vi "create.AddOrderShort.vi"(8 "error in (no error)":errorcluster, 10 "AddOrderShort.Parameters":T1, 11 "AddOrderShort in":refnum<class "AddOrderShort.lvclass">) -> (0 "error out":errorcluster, 3 "AddOrderShort out":refnum<class "AddOrderShort.lvclass">)   [LabVIEW 2020, in "AddOrderShort.lvclass"]
uses:
  AddOrderShort.lvclass
  AddOrderShort.Parameters.ctl
  FieldSpec.ctl
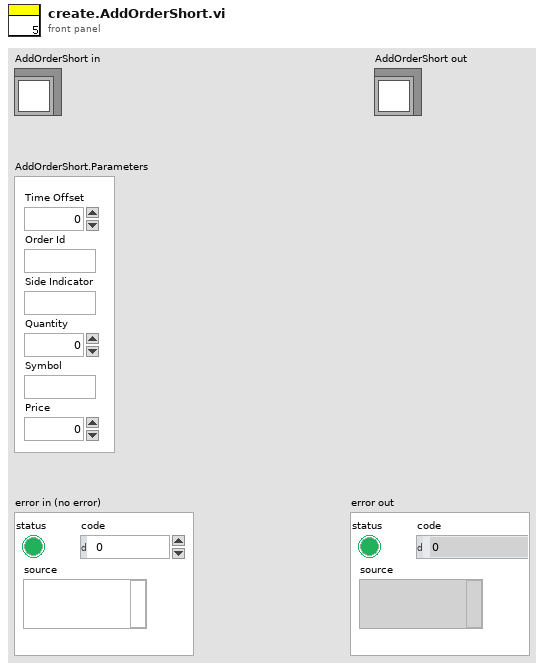
[diagram p1: front panel]
types:
  T1 = typedef "AddOrderShort.lvclass/AddOrderShort.Parameters.ctl" = cluster{"Time Offset":u32, "Order Id":string, "Quantity":u32, "Symbol":string, "Side Indicator":string, "Price":dbl}
  T2 = typedef "FieldSpec.ctl" = cluster{"Name":string, "Offset":i32, "Length":i32, "FieldType":enum16{"Alphanumeric", "Binary", "BinaryLongPrice", "BinaryShortPrice", "BitField", "PrintableAscii", "Value"}, "FieldValue":variant}
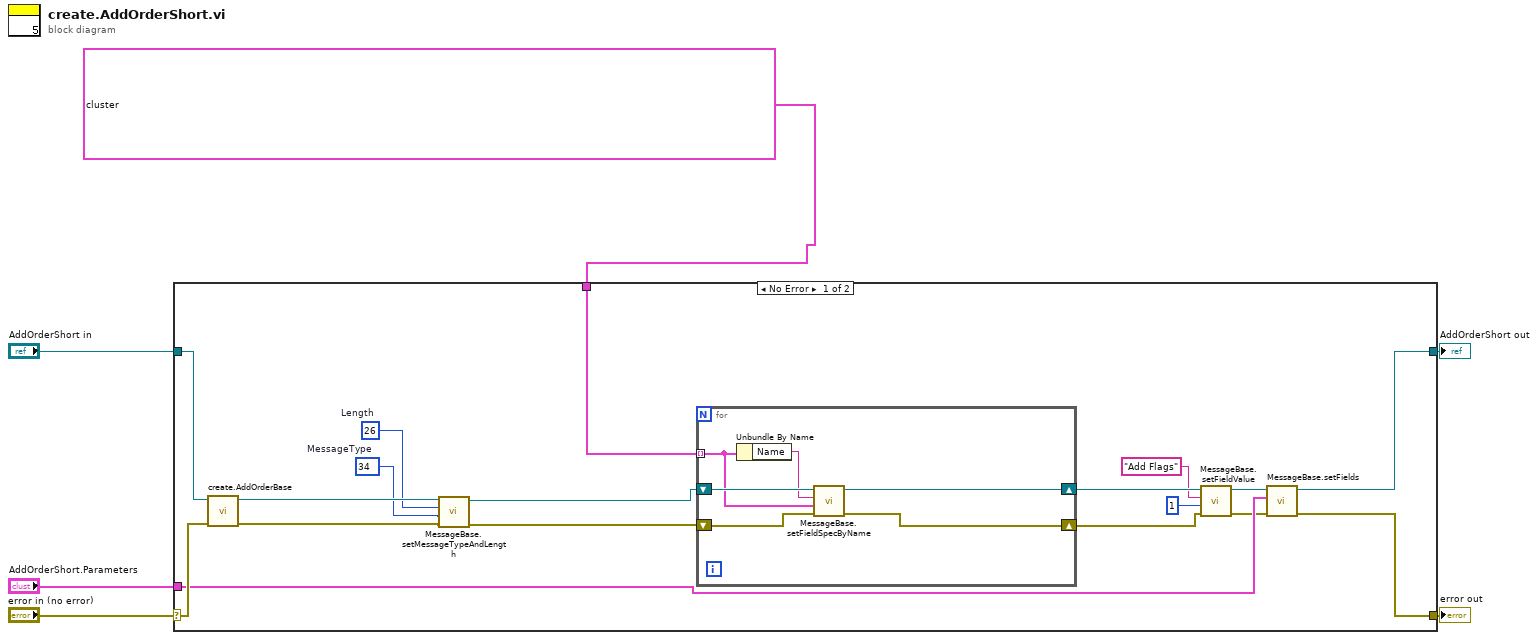
[diagram p0: block diagram]
diagram:
  n1 = case shown="No Error" "error in (no error)" {
    selector: "error in (no error)" -> [w23 w32]
    tunnel: [w14 w32] -> w5
    tunnel: [w13 w31] -> w3
    tunnel: "AddOrderShort in" -> [w24 w31]
    tunnel: T2[] [{"Name"="Quantity", "Offset"=15, "Length"=2, "FieldType"=enum."Binary", "FieldValue"=variant}, {"Name"="Symbol", "Offset"=17, "Length"=6, "FieldType"=enum."PrintableAscii", "FieldValue"=variant}, {"Name"="Price", "Offset"=23, "Length"=2, "FieldType"=enum."BinaryShortPrice", "FieldValue"=variant}, {"Name"="Add Flags", "Offset"=25, "Length"=1, "FieldType"=enum."BitField", "FieldValue"=variant}] ("appended array") -> [w16 _]
    tunnel: "AddOrderShort.Parameters" -> [w15 _]
    frame No Error {
      w21 = u8 34  # MessageType
      w20 = u8 26  # Length
      n2 = call-dynamic "create.AddOrderBase.vi"("error in (no error)"=w23, "AddOrderBase in"=w24) -> ("error out"=w19:errorcluster, "AddOrderBase out"=w22:refnum<class "AddOrderShort.lvclass">)  [unwired: 8 in]
      n3 = call-dynamic "MessageBase.setMessageTypeAndLength.vi"("error in (no error)"=w19, "MessageType"=w21, "Length"=w20, "MessageBase in"=w22) -> ("error out"=w18:errorcluster, "MessageBase out"=w17:refnum<class "AddOrderShort.lvclass">)  [unwired: 6 in]
      n4 = for {
        tunnel: w16 -> [w27] mode=indexing
        shift-right: [w26] -> w10
        shift-left: w17 -> [w30]
        shift-right: [w25] -> w7
        shift-left: w18 -> [w29]
        n5 = Unbundle By Name(w27) -> ("Name"=w28:string)
        n6 = call-dynamic "MessageBase.setFieldSpecByName.vi"("error in (no error)"=w29, "FIeldSpec"=w27, "Field.Name"=w28, "MessageBase in"=w30) -> ("error out"=w25:errorcluster, "MessageBase out"=w26:refnum<class "AddOrderShort.lvclass">)  [unwired: 6 in]
      }
      n7 = call-dynamic "MessageBase.setFieldValue.vi"("error in (no error)"=w7, "Value"=u8 1, "FIeld.Name"="Add Flags", "MessageBase in"=w10) -> ("error out"=w12:errorcluster, "MessageBase out"=w11:refnum<class "AddOrderShort.lvclass">)  [unwired: 6 in]
      n8 = call-dynamic "MessageBase.setFields.vi"("error in (no error)"=w12, "Cluster (dup)"=w15, "MessageBase in"=w11) -> ("error out"=w14:errorcluster, "MessageBase out"=w13:refnum<class "AddOrderShort.lvclass">)  [unwired: 7 in]
    }
    frame Error {
    }
  }
  "error out" <- w5
  "AddOrderShort out" <- w3
